vi "Create_Library_NameMatchesLibraryName.vi"() -> (0 "error out":errorcluster)   [LabVIEW 2019, in "TestSuiteTest.lvlib"]
uses:
  TestSuiteTest.lvlib
  f7b43874-a18c-49d6-a380-8809de24562d.vi
  TestSuite/TestSuite.lvclass
  Constraint/IsEqual/IsEqual.lvclass
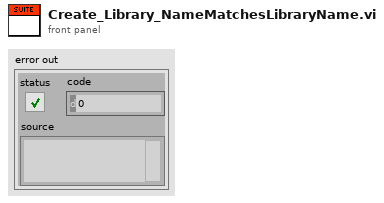
[diagram p1: front panel]
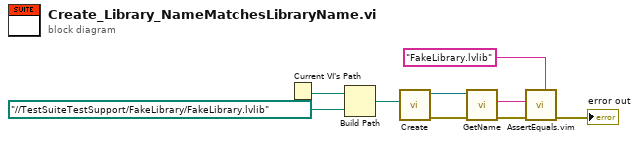
[diagram p0: block diagram]
diagram:
  n1 = Current VI's Path() -> (path=w9:path)
  n2 = Build Path(base path=w9, name or relative path=path "../../TestSuiteTestSupport/FakeLibrary/FakeLibrary.lvlib" ("Path")) -> (appended path=w7:path)
  n3 = call "Create.vi"("Path"=w7) -> ("error out"=w5:errorcluster, "TestSuite"=w6:refnum<class "TestSuite.lvclass">)  [unwired: 9 in]
  n4 = call-dynamic "GetName.vi"("error in (no error)"=w5, "TestSuite in"=w6) -> ("error out"=w4:errorcluster, "Name"=w3:string)  [unwired: 7 in, 1 out]
  n5 = call "AssertEquals.vim"("Expected"="FakeLibrary.lvlib" ("Name"), "error in (no error)"=w4, "Actual"=w3) -> ("error out"=→"error out":errorcluster)  [unwired: 8 in]
